vi "CU_train_NeuralNet.vi"(6 "DataTypes":T1, 8 "error in (no error)":errorcluster, 9 "Indices":i8[](array[numeric]), 10 "# of hidden neuron":i32=10, 11 "ClassifierClass in":refnum<class "ClassifierClass.lvclass">) -> (0 "error out":errorcluster, 1 "exit flag":i32, 2 "ANN out":T2={"Training Data"={"dim in"=0, "dim out"=0, "# samples"=0, "Input"=[], "Output"=[]}, "Normalize Info"={"input min"=[], "input max"=[], "output min"=[], "output max"=[]}, "3-layer NN"={"# input neuron "=0, "# hidden neuron"=0, "# output neuron"=0, "Weight (I->H)"=[], "Weight (H->O)"=[], "Output"=[], "Hidden Out"=[], "Derivation Output"=[], "Derivation Hidden"=[], "dw (I->H)"=[], "dw (H->O)"=[]}, "Ternimal Condition"={"min MSE"=1e-05, "min delta MSE"=1e-05, "min step length"=1e-08, "max iteration"=inf}}, 3 "ClassifierClass out":refnum<class "ClassifierClass.lvclass">)   [LabVIEW 2016, in "Classifier.lvlib" / "ClassifierClass.lvclass"]
uses:
  ClassifierClass.lvclass
  <vilib>/addons/Machine Learning/Supervised Learning/ml_BP_Project.ctl
  <vilib>/addons/Machine Learning/Supervised Learning/ml_BP_Data.ctl
  <vilib>/addons/Machine Learning/Supervised Learning/ml_BP_Normalize Data.ctl
  <vilib>/addons/Machine Learning/Supervised Learning/ml_BP_3layer Feedforward.ctl
  <vilib>/addons/Machine Learning/Supervised Learning/ml_BP_Terminal Condition.ctl
  CU_DataTypes.ctl
  ClassifierClass.lvclass/ClassifierClass.ctl
  <vilib>/addons/Machine Learning/NILabs_MLT.lvlib
  Classifier.lvlib
panel:
  # "This VI is a part of BCI Design library, http://www.ru-bci.org \nCopyright © 2020, Sotnikov Peter, All rights reserved. License: GNU GPLv3"
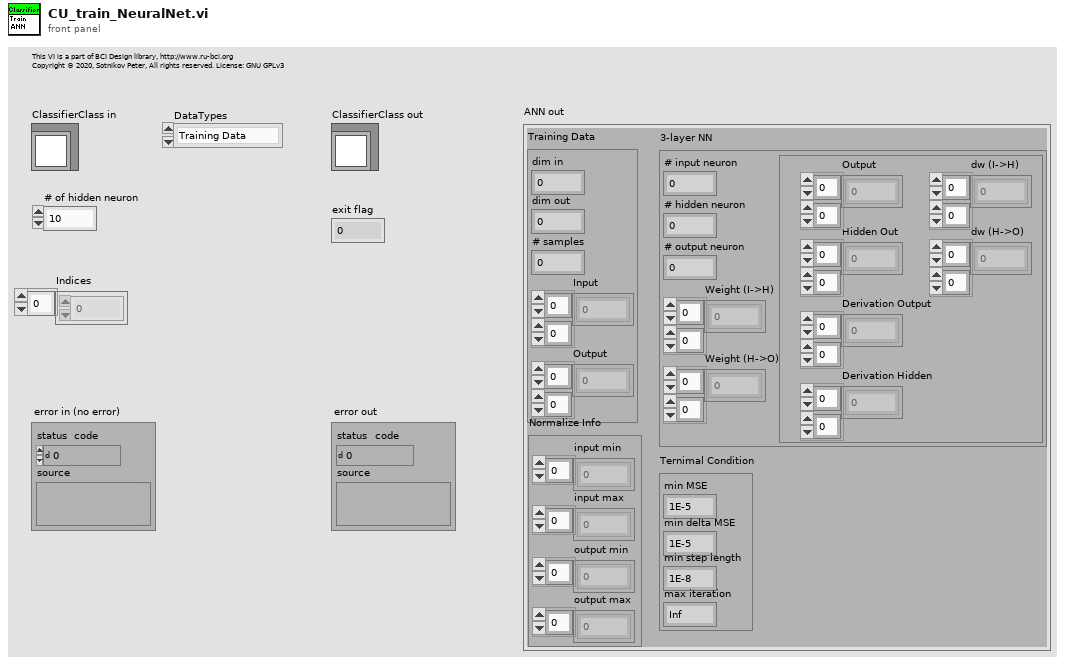
[diagram p1: front panel]
types:
  T1 = typedef "Classifier.lvlib/CU_DataTypes.ctl" = enum16{"Training Data", "Test Data", "Training Data (cross-check)", "Test Data (cross-check)"}
  T2 = typedef "NILabs_MLT.lvlib/ml_BP_Project.ctl" = cluster{"Training Data":T3, "Normalize Info":T4, "3-layer NN":T5, "Ternimal Condition":T6}
  T3 = typedef "NILabs_MLT.lvlib/ml_BP_Data.ctl" = cluster{"dim in":i32, "dim out":i32, "# samples":i32, "Input":dbl[][], "Output":dbl[][]}
  T4 = typedef "NILabs_MLT.lvlib/ml_BP_Normalize Data.ctl" = cluster{"input min":dbl[], "input max":dbl[], "output min":dbl[], "output max":dbl[]}
  T5 = typedef "NILabs_MLT.lvlib/ml_BP_3layer Feedforward.ctl" = cluster{"# input neuron ":i32, "# hidden neuron":i32, "# output neuron":i32, "Weight (I->H)":dbl[][], "Weight (H->O)":dbl[][], "Output":dbl[][], "Hidden Out":dbl[][], "Derivation Output":dbl[][], "Derivation Hidden":dbl[][], "dw (I->H)":dbl[][], "dw (H->O)":dbl[][]}
  T6 = typedef "NILabs_MLT.lvlib/ml_BP_Terminal Condition.ctl" = cluster{"min MSE":dbl, "min delta MSE":dbl, "min step length":dbl, "max iteration":dbl}
  T7 = typedef "XML_EEG_Features.lvlib/XML_FF_Trial.ctl" = cluster{"ClassLabel":string, "FeatureVector":dbl[]}
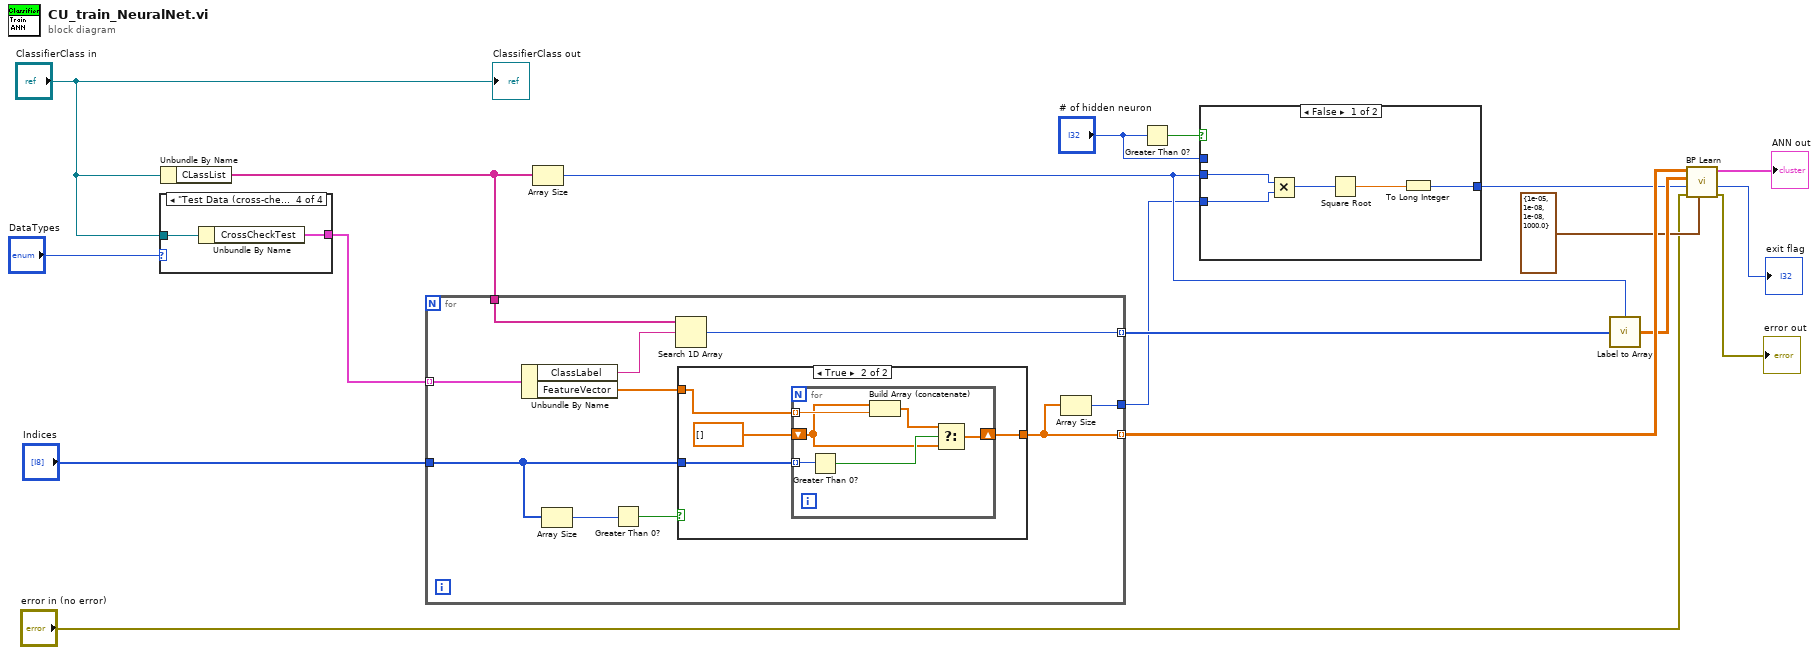
[diagram p0: block diagram]
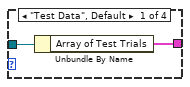
[diagram p2: hidden frame]
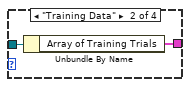
[diagram p3: hidden frame]
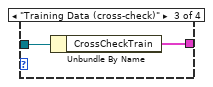
[diagram p4: hidden frame]
diagram:
  n1 = case shown="\"Test Data (cross-check)\"" "DataTypes" {
    tunnel: "ClassifierClass in" -> [w20 w22 w24 w26]
    tunnel: [w19 w21 w23 w25] -> w7
    frame "Test Data", Default {
      n2 = Unbundle By Name(w20) -> ("Array of Test Trials"=w19:T7[])
    }
    frame "Training Data" {
      n3 = Unbundle By Name(w22) -> ("Array of Training Trials"=w21:T7[])
    }
    frame "Training Data (cross-check)" {
      n4 = Unbundle By Name(w24) -> ("CrossCheckTrain"=w23:T7[])
    }
    frame "Test Data (cross-check)" {
      n5 = Unbundle By Name(w26) -> ("CrossCheckTest"=w25:T7[])
    }
  }
  n6 = Unbundle By Name("ClassifierClass in") -> ("CLassList"=w5:string[])
  n7 = for {
    tunnel: w7 -> [w36] mode=indexing
    tunnel: "Indices" -> [w32]
    tunnel: w5 -> [w31]
    tunnel: [w29] -> w17 mode=indexing
    tunnel: [w28] -> w16 mode=indexing
    tunnel: [w27] -> w2
    n8 = Unbundle By Name(w36) -> ("ClassLabel"=w30:string, "FeatureVector"=w33:dbl[])
    n9 = Array Size(array=w32) -> (size(s)=w35:i32)
    n10 = Greater Than 0?(x=w35) -> (x > 0?=w34:bool)
    n11 = Search 1D Array(1D array=w31, element=w30) -> (index of element=w29:i32)  [unwired: 1 in]
    n12 = case shown="True" w34 {
      tunnel: w33 -> [w37 w41]
      tunnel: [w37 w38] -> w28
      tunnel: w32 -> [_ w40]
      frame False {
      }
      frame True {
        n13 = for {
          tunnel: w41 -> [w44] mode=indexing
          tunnel: w40 -> [w47] mode=indexing
          shift-right: [w46] -> w38
          shift-left: dbl[] [] -> [w42]
          n14 = Greater Than 0?(x=w47) -> (x > 0?=w45:bool)
          n15 = Build Array (concatenate)(w42, w44) -> (w43:dbl[])
          n16 = Select(t=w43, s=w45, f=w42) -> (s? t:f=w46:dbl[])
        }
      }
    }
    n17 = Array Size(array=w28) -> (size(s)=w27:i32)
  }
  n18 = Array Size(array=w5) -> (size(s)=w3:i32)
  n19 = Greater Than 0?(x="# of hidden neuron") -> (x > 0?=w10:bool)
  n20 = case shown="False" w10 {
    tunnel: [w51 w53] -> w4
    tunnel: "# of hidden neuron" -> [_ w53]
    tunnel: w3 -> [w49 _]
    tunnel: w2 -> [w48 _]
    frame False {
      n21 = Multiply(x=w49, y=w48) -> (x*y=w52:i32)
      n22 = Square Root(x=w52) -> (sqrt(x)=w50:dbl)
      n23 = To Long Integer(number=w50) -> (32bit integer=w51:i32)
    }
    frame True {
    }
  }
  n24 = call <vilib>:"Label to Array.vi"("Classes"=w17, "# of classes"=w3) -> ("Array"=w15:dbl[][])
  n25 = call <vilib>:"BP Learn.vi"("Stopping Criteria"=T6 {"min MSE"=1e-05, "min delta MSE"=1e-08, "min step length"=1e-08, "max iteration"=1000.0}, "error in (no error)"="error in (no error)", "# of hidden neuron"=w4, "Training outputs"=w15, "Training data samples"=w16) -> ("error out"=→"error out":errorcluster, "exit flag"=→"exit flag":i32, "BP Project"=→"ANN out":T2)  [unwired: 3 in, 1 out]
  "ClassifierClass out" <- "ClassifierClass in"
